vi "CreatePublicEvents.vi"(8 "error in (no error)":errorcluster, 11 "Home":refnum<class "Home.lvclass">) -> (0 "error out":errorcluster, 3 "Home out":refnum<class "Home.lvclass">)   [LabVIEW 2022 SP3, in "Home.lvclass"]
uses:
  Home.lvclass
  Home.lvclass/Home.ctl
  Typedefs/Home State--enum.ctl
  <vilib>/JKI/JKI SMO/SMO/SMO.lvclass
panel:
  # "For instructions on how to use the JKI State Machine Objects, examples and video tutorials, visit:\nhttp://jki.net/state-machine-objects/\n\nJKI State Machine Objects™\nhttp://jki.net/state-machine-objects/\nCopyright (C) 2005-2015, JKI <info@jki.net>\nALL RIGHTS RESERVED"
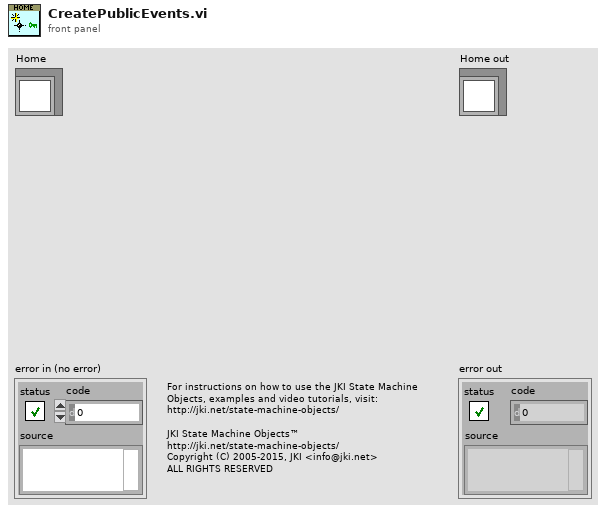
[diagram p1: front panel]
types:
  T1 = typedef "Home.lvclass/Home State--enum.ctl" = enum16{"unknown", "Opened", "Embedded", "Closed"}
  T2 = typedef "Home.lvclass/PrivateData--Ref.ctl" = refnum<data-value>
  T3 = typedef "Home.lvclass/PrivateData--Cluster.ctl" = cluster{"Public Events":T4, "Subpanel Ref":refnum<vi>, "UI State":T5}
  T4 = typedef "Home.lvclass/PublicEvents--Cluster.ctl" = cluster{"UI State":refnum<user-event>}
  T5 = typedef "Home.lvclass/SMO.UI_Embed State--enum.ctl" = enum16{"unknown", "Opened", "Embedded", "Closed"}
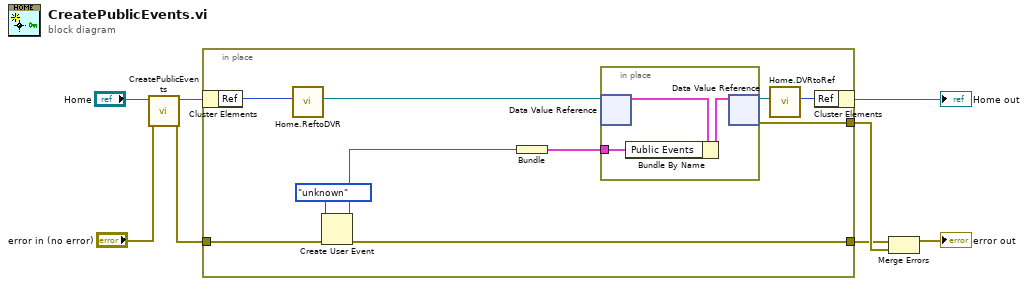
[diagram p0: block diagram]
diagram:
  n1 = call-parent "CreatePublicEvents.vi"("error in (no error)"="error in (no error)", "SMO"="Home") -> ("error out"=w2:errorcluster, "SMO out"=w3:refnum<class "Home.lvclass">)  [unwired: 8 in]
  n2 = in-place {
    in-place-border: [w18] -> w8
    in-place-border: w2 -> [w9]
    in-place-border: [w12] -> w1
    n3 = in-place-cluster #1(w3) -> ("Ref"=w17:u32)
    n4 = call "Home.ReftoDVR.vi"("Ref"=w17) -> ("Ref"=w16:T2)  [unwired: 10 in]
    n5 = Create User Event(user event datatype=Home_State--enum."unknown" ("UI State"), error in=w9) -> (user event=w11:refnum<user-event>, error out=w12:errorcluster)
    n6 = Bundle("UI State"=w11) -> (w15:cluster{"UI State":refnum<user-event>})  [unwired: 1 in]
    n7 = in-place {
      in-place-border: w15 -> [w19]
      n8 = in-place-dvr #2(w16) -> (w21:T3)  [unwired: 1 out]
      n9 = Bundle By Name(cluster=w21, "Public Events"=w19) -> (w20:T3)
      n10 = in-place-dvr #2(w20) -> (w14:T2, w18:errorcluster)
    }
    n11 = call "Home.DVRtoRef.vi"("Ref"=w14) -> ("Ref"=w13:u32)  [unwired: 10 in]
    n12 = in-place-cluster #1("Ref"=w13) -> (→"Home out":refnum<class "Home.lvclass">)
  }
  n13 = Merge Errors(w1, w8) -> (→"error out":errorcluster)
